vi "RCM_Write JPG File.vi"(5 "quality (80)":i32=80, 8 "error in (no error)":errorcluster, 10 "image data":T1) -> (0 "error out":errorcluster)   [LabVIEW 2014]
uses:
  <vilib>/picture/picture.llb/imagedata.ctl
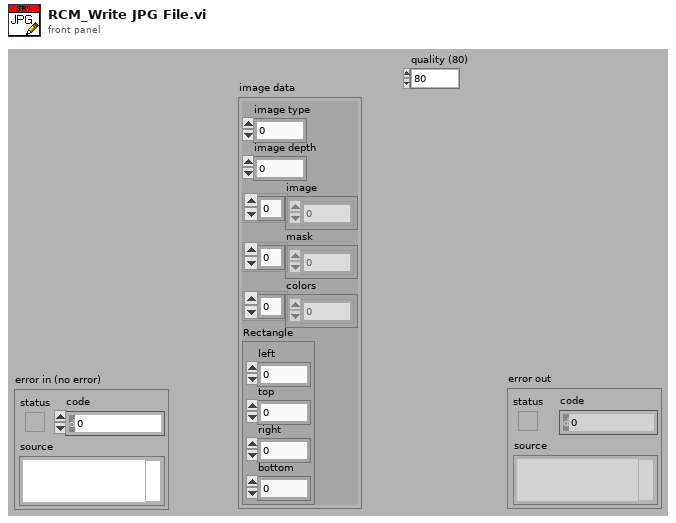
[diagram p1: front panel]
types:
  T1 = typedef "imagedata.ctl" = cluster{"image type":i32, "image depth":i32, "image":u8[], "mask":u8[], "colors":u32[], "Rectangle":cluster{"left":i16, "top":i16, "right":i16, "bottom":i16}}
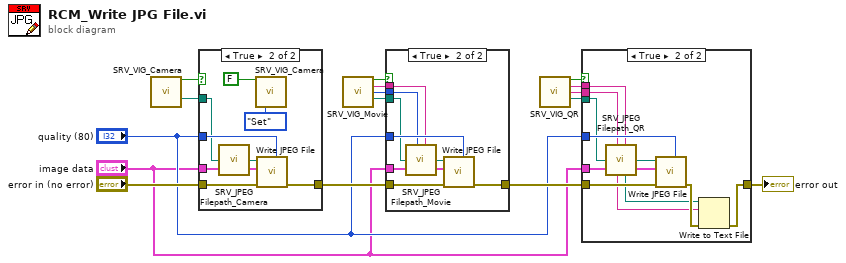
[diagram p0: block diagram]
diagram:
  n1 = call "SRV_VIG_Camera.vi"() -> ("Camera?"=w10:bool, "Images Directory Path out"=w9:path)  [unwired: 14 in]
  n2 = case shown="True" w10 {
    tunnel: "image data" -> [_ w25]
    tunnel: "error in (no error)" -> [w17 w24]
    tunnel: [w17 w23] -> w15
    tunnel: "quality (80)" -> [_ w22]
    tunnel: w9 -> [_ w18]
    frame False {
    }
    frame True {
      n3 = call "SRV_JPEG Filepath_Camera.vi"("Dir path for JPEG file"=w18) -> ("JPEG Filepath"=w20:path)  [unwired: 8 in]
      n4 = call "SRV_VIG_Camera.vi"("Camera"=FALSE, "Method (Get)"=enum16{"Get", "Set"}."Set") -> ()  [unwired: 12 in, 2 out]
      n5 = call <vilib>:"Write JPEG File.vi"("quality (80)"=w22, "error in (no error)"=w24, "image data"=w25, "path to JPEG file"=w20) -> ("error out"=w23:errorcluster)  [unwired: 6 in, 1 out]
    }
  }
  n6 = call "SRV_VIG_Movie.vi"() -> ("Movie?"=w14:bool, "Timestamp String out"=w13:string, "Count out"=w12:i32, "Images Directory Path out"=w11:path)  [unwired: 12 in]
  n7 = case shown="True" w14 {
    tunnel: "image data" -> [_ w34]
    tunnel: "quality (80)" -> [_ w33]
    tunnel: w15 -> [w26 w32]
    tunnel: [w26 w31] -> w8
    tunnel: w13 -> [_ w29]
    tunnel: w12 -> [_ w28]
    tunnel: w11 -> [_ w27]
    frame False {
    }
    frame True {
      n8 = call "SRV_JPEG Filepath_Movie.vi"("Count"=w28, "Dir path for JPEG file"=w27, "Timestamp String"=w29) -> ("JPEG Filepath"=w30:path)  [unwired: 6 in]
      n9 = call <vilib>:"Write JPEG File.vi"("quality (80)"=w33, "error in (no error)"=w32, "image data"=w34, "path to JPEG file"=w30) -> ("error out"=w31:errorcluster)  [unwired: 6 in, 1 out]
    }
  }
  n10 = call "SRV_VIG_QR.vi"() -> ("QR?"=w4:bool, "Timestamp String out"=w3:string, "QR Code out"=w1:string, "Images Directory Path out"=w2:path)  [unwired: 12 in]
  n11 = case shown="True" w4 {
    tunnel: "image data" -> [_ w45]
    tunnel: "quality (80)" -> [_ w44]
    tunnel: w8 -> [w35 w43]
    tunnel: [w35 w36] -> w7
    tunnel: w3 -> [_ w41]
    tunnel: w2 -> [_ w40]
    tunnel: w1 -> [_ w39]
    frame False {
    }
    frame True {
      n12 = call "SRV_JPEG Filepath_QR.vi"("QR Code"=w39, "Dir path for JPEG file"=w40, "Timestamp String"=w41) -> ("QR Code dup"=w38:string, "QR JPEG Filepath"=w42:path, "QR Text Filepath"=w37:path)  [unwired: 4 in]
      n13 = call <vilib>:"Write JPEG File.vi"("quality (80)"=w44, "error in (no error)"=w43, "image data"=w45, "path to JPEG file"=w42) -> ("error out"=w46:errorcluster)  [unwired: 6 in, 1 out]
      n14 = Write to Text File(file (use dialog)=w37, text=w38, error in=w46) -> (error out=w36:errorcluster)  [unwired: 1 in, 2 out]
    }
  }
  "error out" <- w7
